vi "Pressure Unit.vi"(7 "Set? (F:Read)":bool, 8 "Error In":errorcluster, 9 "Unit (Pa)":T1(ring)=enum."1.0000 Pa", 11 "VISA resource name":refnum<visa-resource-name>) -> (0 "Error Out":errorcluster, 1 "Unit (Pa)":T1(ring)=enum."1.0000 Pa", 3 "dup VISA resource name":refnum<visa-resource-name>)   [LabVIEW 2011, in "MGC647C.lvlib"]
doc: "Read/set pressure unit."
uses:
  <instrlib>/MGC647C/MGC647C.lvlib
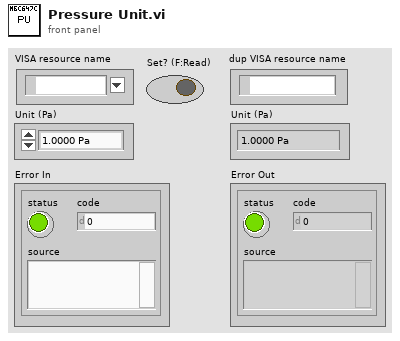
[diagram p1: front panel]
types:
  T1 = enum16{"1.0000 mTorr", "10.000 mTorr", "100.00 mTorr", "1000.0 mTorr", "1.0000 Torr", "10.000 Torr", "100.00 Torr", "1000.0 Torr", "1.0000 kTorr", "10.000 kTorr", "100.00 kTorr", "1.0000 µBar", "10.000 µBar", "100.00 µBar", "1000.0 µBar", "1.0000 mBar", "10.000 mBar", "100.00 mBar", "1000.0 mBar", "1.0000 Bar", "10.000 Bar", "100.00 Bar", "1.0000 Pa", "10.000 Pa", "100.00 Pa", "1.0000 kPa", "10.000 kPa", "100.00 kPa", "1000.0 kPa", "2.0000 mTorr", "5.0000 mTorr", "20.000 mTorr", "50.000 mTorr", "200.00 mTorr", "500.00 mTorr", "2000.0 mTorr", "5000.0 mTorr", "2.0000 Torr", "5.0000 Torr", "20.000 Torr", "50.000 Torr", "200.00 Torr", "500.00 Torr", "2000.0 Torr", "5000.0 Torr", "2.0000 kTorr", "5.0000 kTorr", "20.000 kTorr", "50.000 kTorr", "2.0000 µbar", "5.0000 µbar", "20.000 µbar", "50.000 µbar", "200.00 µbar", "500.00 µbar", "2000.0 µbar", "5000.0 µbar", "2.0000 mbar", "5.0000 mbar", "20.000 mbar", "50.000 mbar", "200.00 mbar", "500.00 mbar", "2000.0 mbar", "5000.0 mbar", "2.0000 bar", "5.0000 bar", "20.000 bar", "50.000 bar", "2.0000 Pa", "5.0000 Pa", "20.000 Pa", "50.000 Pa", "200.00 Pa", "500.00 Pa", "2.0000 kPa", "5.0000 kPa", "20.000 kPa", "50.000 kPa", "200.00 kPa", "500.00 kPa", "2000.0 kPa", "5000.0 kPa", "1.0000 MPa", "2.0000 MPa", "5.0000 MPa", "10.000 MPa"}
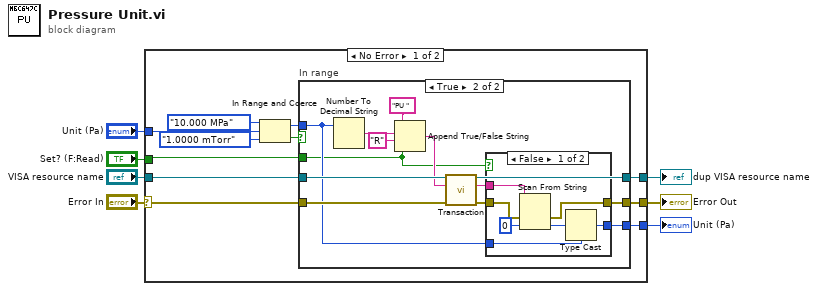
[diagram p0: block diagram]
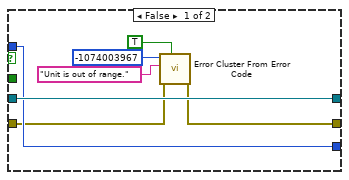
[diagram p2: hidden frame]
diagram:
  n1 = case shown="No Error" "Error In" {
    selector: "Error In" -> [w12 w49]
    tunnel: "VISA resource name" -> [w18 w48]
    tunnel: [w17 w48] -> w6
    tunnel: [w16 w49] -> w5
    tunnel: "Set? (F:Read)" -> [w15 _]
    tunnel: "Unit (Pa)" -> [w14 w50]
    tunnel: [w11 w50] -> w1
    frame No Error {
      n2 = In Range and Coerce(upper limit=T1."10.000 MPa", x=w14, lower limit=T1."1.0000 mTorr") -> (coerced(x)=w13:T1, In Range?=w10:bool)
      n3 = case "In range" shown="True" w10 {
        tunnel: w18 -> [w25 w38]
        tunnel: [w25 w37] -> w17
        tunnel: [w19 w36] -> w16
        tunnel: w15 -> [_ w26]
        tunnel: w13 -> [w24 w27]
        tunnel: w12 -> [w20 w35]
        tunnel: [w24 w28] -> w11
        frame False {
          n4 = call <vilib>:"Error Cluster From Error Code.vi"("show call chain? (False)"=TRUE, "error in (no error)"=w20, "error message (\"\")"="Unit is out of range." ("error message (\"\")"), "error code (0)"=-1074003967) -> ("error out"=w19:errorcluster)  [unwired: 5 in]
        }
        frame True {
          n5 = Number To Decimal String(number=w27) -> (decimal integer string=w29:string)  [unwired: 1 in]
          n6 = Append True/False String(1:w26, 2:"R" ("false string"), 3:w29, 4:"PU " ("string (\"\")")) -> (0:w30:string)
          n7 = call <instrlib>:"Transaction.vi"("Error In"=w35, "Command"=w30, "VISA resource name"=w38) -> ("Error Out"=w31:errorcluster, "Response"=w32:string, "dup VISA resource name"=w37:refnum<visa-resource-name>)  [unwired: 6 in]
          n8 = case shown="False" w26 {
            tunnel: [w45 w47] -> w36
            tunnel: w32 -> [w44 _]
            tunnel: w31 -> [w43 w47]
            tunnel: [w41 w46] -> w28
            tunnel: w27 -> [w40 w46]
            frame False {
              n9 = Scan From String(input string=w44, error in=w43, default 1=u16 0 ("default value 1")) -> (error out=w45:errorcluster, output 1=w42:u16)  [unwired: 2 in, 2 out]
              n10 = Type Cast(type=w40, x=w42) -> (*(type *) &x=w41:T1)
            }
            frame True {
            }
          }
        }
      }
    }
    frame Error {
    }
  }
  "dup VISA resource name" <- w6
  "Error Out" <- w5
  "Unit (Pa)" <- w1
